vi "Wmeter Initialize.vi"(8 "error in":errorcluster, 11 "Serial Settings":T1={"VISA resource name"="COM6", "baud rate"=9600, "data bits"=8, "parity"=0, "stop bits"=10, "flow control"=2, "termination char\n(0xA = '\\n' = LF)"=10, "timeout (ms)"=1000, "End write with termination character?"=TRUE, "End read on termination character?"=TRUE} {"termination char\n(0xA = '\\n' = LF)" format="%.0x"; "flow control" items=["None"=0, "XON/XOFF"=1, "RTS/CTS"=2, "DTR/DSR"=4]; "stop bits" items=["1.0"=10, "1.5"=15, "2.0"=20]; "parity" items=["None", "Odd", "Even", "Mark", "Space"]; "data bits" min=5 max=8 step=1}) -> (0 "error out (no error)":errorcluster, 3 "VISA RName out":refnum<visa-resource-name>)   [LabVIEW 2012]
uses:
  <vilib>/Instr/_visa.llb/VISA Configure Serial Port (Instr).vi
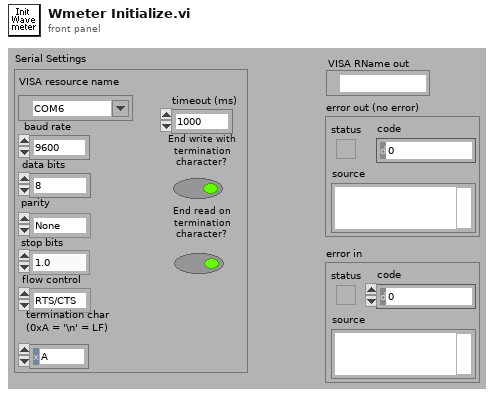
[diagram p1: front panel]
types:
  T1 = cluster{"VISA resource name":refnum<visa-resource-name>, "baud rate":u32, "data bits":u16, "parity":u16, "stop bits":u16, "flow control":u16, "termination char\n(0xA = '\\n' = LF)":u8, "timeout (ms)":u32, "End write with termination character?":bool, "End read on termination character?":bool}
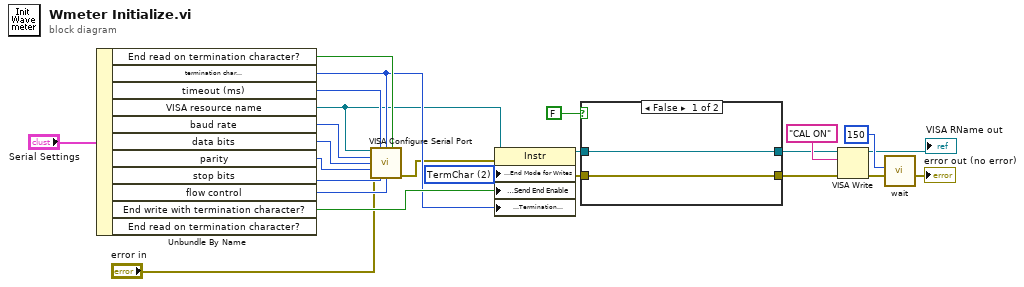
[diagram p0: block diagram]
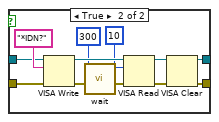
[diagram p2: hidden frame]
diagram:
  w14 = u16 2 items=["None", "LastBit", "TermChar", "Break"] ("Serial Settings:Serial End Mode for Writes")
  n1 = Unbundle By Name("Serial Settings") -> ("End read on termination character?"=w17:bool, "termination char\n(0xA = '\\n' = LF)"=w15:u8, "timeout (ms)"=w18:u32, "VISA resource name"=w13:refnum<visa-resource-name>, "baud rate"=w23:u32, "data bits"=w22:u16, "parity"=w21:u16, "stop bits"=w20:u16, "flow control"=w19:u16, "End write with termination character?"=w16:bool)  [unwired: 1 out]
  n2 = call-poly "VISA Configure Serial Port"("VISA resource name"=w13, "timeout (10sec)"=w18, "termination char\n(0xA = '\\n' = LF)"=w15, "Enable Termination\nChar (T)"=w17, "baud rate (9600)"=w23, "data bits (8)"=w22, "parity (0:none)"=w21, "error in (no error)"="error in", "stop bits (10: 1 bit)"=w20, "flow control (0:none)"=w19) -> ("error out"=w12:errorcluster)  [unwired: 4 in, 1 out]
  n3 = property class="Instr"(reference=w13, error in=w12, "Serial Settings:End Mode for Writes"=w14, "Message Based Settings:Send End Enable"=w16, "Message Based Settings:Termination Character"=w15) -> (reference out=w6:refnum<visa-resource-name>, error out=w7:errorcluster)
  n4 = case shown="False" FALSE {
    tunnel: w7 -> [w25 w35]
    tunnel: w6 -> [w26 w34]
    tunnel: [w26 w31] -> w5
    tunnel: [w25 w30] -> w4
    frame False {
    }
    frame True {
      n5 = VISA Write(VISA resource name=w34, write buffer="*IDN?" ("data"), error in (no error)=w35) -> (VISA resource name out=w37:refnum<visa-resource-name>, error out=w29:errorcluster)  [unwired: 1 out]
      n6 = call "wait.vi"("error in (no error)"=w29, "ms to wait"=u32 300) -> ("error out (no error)"=w28:errorcluster)  [unwired: 7 in]
      n7 = VISA Read(VISA resource name=w37, byte count=10, error in (no error)=w28) -> (VISA resource name out=w33:refnum<visa-resource-name>, error out=w32:errorcluster)  [unwired: 2 out]
      n8 = VISA Clear(VISA resource name=w33, error in (no error)=w32) -> (VISA resource name out=w31:refnum<visa-resource-name>, error out=w30:errorcluster)
    }
  }
  n9 = VISA Write(VISA resource name=w5, write buffer="CAL ON" ("data"), error in (no error)=w4) -> (VISA resource name out=→"VISA RName out":refnum<visa-resource-name>, error out=w11:errorcluster)  [unwired: 1 out]
  n10 = call "wait.vi"("error in (no error)"=w11, "ms to wait"=u32 150) -> ("error out (no error)"=→"error out (no error)":errorcluster)  [unwired: 7 in]
